vi "updateEndTime.vi"(8 "error in (no error)":errorcluster, 11 "RfRamp in":refnum<class "RfRamp.lvclass">) -> (0 "error out":errorcluster, 3 "RfRamp out":refnum<class "RfRamp.lvclass">)   [LabVIEW 2009, in "Tools.lvlib" / "Scripting.lvlib" / "RfRamp.lvclass"]
uses:
  RfRamp.lvclass
  RfRamp.lvclass/RfRamp.ctl
  ScriptEvent.lvclass
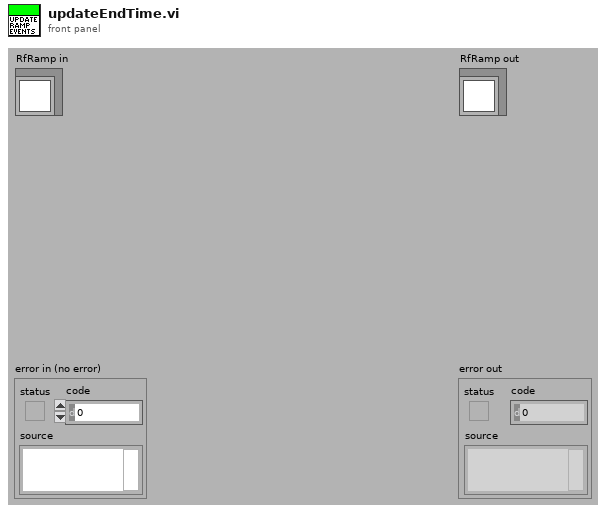
[diagram p1: front panel]
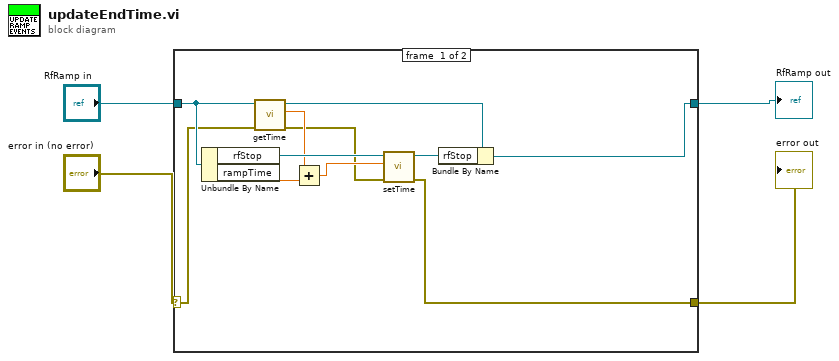
[diagram p0: block diagram]
diagram:
  n1 = case shown="No Error" "error in (no error)" {
    selector: "error in (no error)" -> [w6 w16]
    tunnel: [w7 w17] -> w4
    tunnel: "RfRamp in" -> [w14 w17]
    tunnel: [w5 w16] -> w1
    frame #0 {
      n2 = Unbundle By Name(w14) -> ("rfStop"=w15:refnum<class "rf.lvclass">, "rampTime"=w11:dbl)
      n3 = call "getTime.vi"("error in (no error)"=w6, "ScriptEvent.lvclass in"=w14) -> ("error out"=w10:errorcluster, "time"=w13:dbl, "ScriptEvent.lvclass out"=w9:refnum<class "RfRamp.lvclass">)  [unwired: 7 in]
      n4 = Add(x=w13, y=w11) -> (x+y=w12:dbl)
      n5 = call "setTime.vi"("error in (no error)"=w10, "time"=w12, "ScriptEvent.lvclass in"=w15) -> ("error out"=w5:errorcluster, "ScriptEvent.lvclass out"=w8:refnum<class "rf.lvclass">)  [unwired: 7 in]
      n6 = Bundle By Name(cluster=w9, "rfStop"=w8) -> (w7:refnum<class "RfRamp.lvclass">)
    }
    frame #1 {
    }
  }
  "error out" <- w1
  "RfRamp out" <- w4
